vi "TDMS_Init.vi"(0 "object in":refnum<class "TDMS.lvclass">, 2 "Data Method":refnum<class "IDataMethod.lvclass">, 5 "error in (no error)":errorcluster) -> (14 "object out":refnum<class "TDMS.lvclass">, 19 "error out":errorcluster)   [LabVIEW 2024, in "TDMS.lvclass"]
uses:
  TDMS.lvclass
  C:/Users/burakkorkmaz/Desktop/Leveling/labview-desing-patterns/Bridge Pattern/Abstractions/DataType/DataType.lvclass
  TDMS.lvclass/TDMS.ctl
  DataType/DataType.lvclass
  C:/Users/burakkorkmaz/Desktop/Leveling/labview-desing-patterns/Bridge Pattern/Abstractions/TDMS/TDMS.lvclass
  IDataMethod_interface/IDataMethod.lvclass
panel:
  # "Connector Pane"
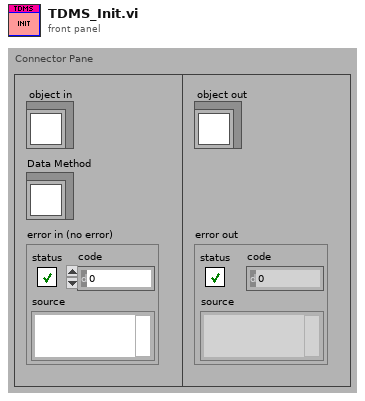
[diagram p1: front panel]
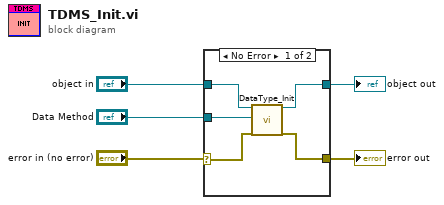
[diagram p0: block diagram]
diagram:
  n1 = case shown="No Error" "error in (no error)" {
    selector: "error in (no error)" -> [w10 w11]
    tunnel: [w7 w12] -> w5
    tunnel: "object in" -> [w8 w12]
    tunnel: [w9 w11] -> w2
    tunnel: "Data Method" -> [w6 _]
    frame No Error {
      n2 = call "DataType_Init.vi"("object in"=w8, "Data Method"=w6, "error in (no error)"=w10) -> ("object out"=w7:refnum<class "TDMS.lvclass">, "error out"=w9:errorcluster)  [unwired: 15 in]
    }
    frame Error {
    }
  }
  "object out" <- w5
  "error out" <- w2
